vi "ModifyingMyAttribute.vi"(0 "reference in":refnum<class "MyG#G3Templ.lvclass">, 2 "increment":dbl, 5 "error in (no error)":errorcluster) -> (14 "reference out":refnum<class "MyG#G3Templ.lvclass">, 19 "error out":errorcluster)   [LabVIEW 2020, in "MyG#G3Templ.lvclass"]
uses:
  MyG#G3Templ.lvclass
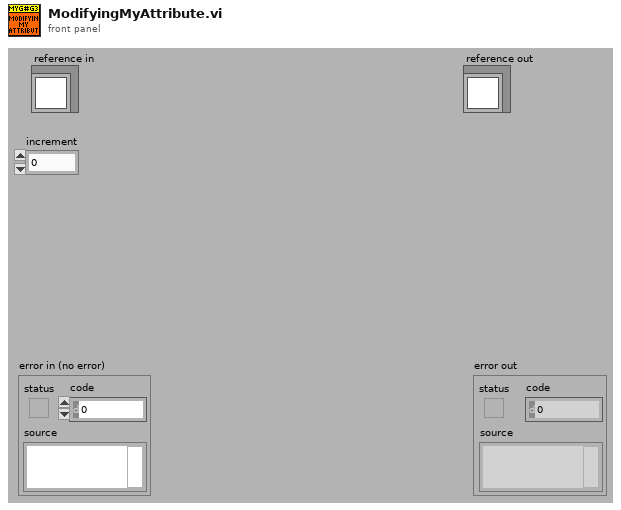
[diagram p1: front panel]
types:
  T1 = typedef "MyG#G3Templ.lvclass/ObjectAttributes.ctl" = cluster{"MyAttribute":dbl}
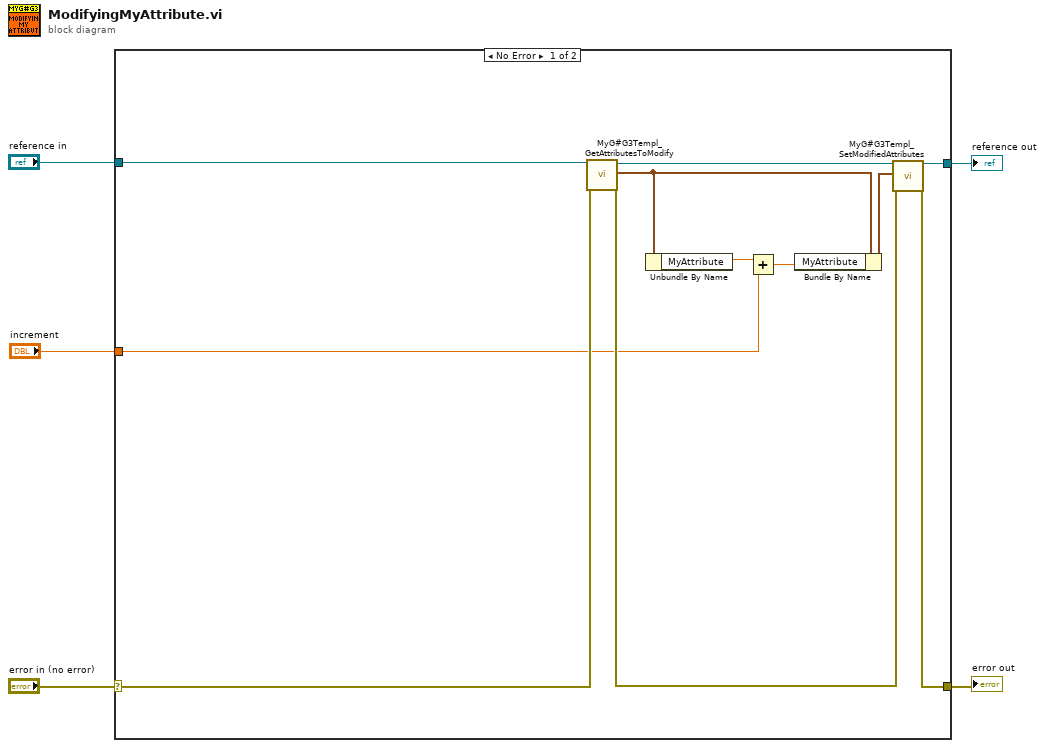
[diagram p0: block diagram]
diagram:
  n1 = case shown="No Error" "error in (no error)" {
    selector: "error in (no error)" -> [w12 w18]
    tunnel: [w14 w18] -> w4
    tunnel: [w11 w17] -> w2
    tunnel: "reference in" -> [w13 w17]
    tunnel: "increment" -> [w6 _]
    frame No Error {
      n2 = call "MyG#G3Templ_GetAttributesToModify.vi"("reference in"=w13, "error in (no error)"=w12) -> ("reference out"=w15:refnum<class "MyG#G3Templ.lvclass">, "attributes"=w9:T1, "error out"=w10:errorcluster)  [unwired: 13 in, 2 out]
      n3 = Unbundle By Name(w9) -> ("MyAttribute"=w8:dbl)
      n4 = Add(x=w8, y=w6) -> (x+y=w7:dbl)
      n5 = Bundle By Name(cluster=w9, "MyAttribute"=w7) -> (w16:T1)
      n6 = call "MyG#G3Templ_SetModifiedAttributes.vi"("reference in"=w15, "attributes"=w16, "error in (no error)"=w10) -> ("reference out"=w11:refnum<class "MyG#G3Templ.lvclass">, "error out"=w14:errorcluster)  [unwired: 15 in]
    }
    frame Error {
    }
  }
  "error out" <- w4
  "reference out" <- w2
